vi "Update_Caliper_Overlay.vi"(5 "Analysis_Point_Result":T1[](array[typedef]), 7 "CaliperEntry":T3 {"CaliperType" items=["Distance", "Mid Point", "Perpendicular Projection", "Lines Intersection", "Angle from Horizontal", "Angle from Vertical", "Angle Defined by 3 Points", "Angle Defined by 4 Points", "Bissecting Line", "Mid Line", "Center of Mass", "Area", "Line Fit", "Circle Fit", "Ellipse Fit"]}, 11 "Image Refnum":refnum<vi>) -> ()   [LabVIEW 2019]
uses:
  Caliper/Controls/CaliperDataEntry.ctl
  Caliper/Controls/CaliperType.ctl
  Caliper/Controls/SelectionListEntry.ctl
  Caliper/Controls/SelectionListEntryPointType.ctl
  Caliper/Controls/CaliperResult.ctl
  Analysis/Controls/Analysis_Result_To_Caliper.ctl
panel:
  in  "Vision_Image":T2(plugin-control)
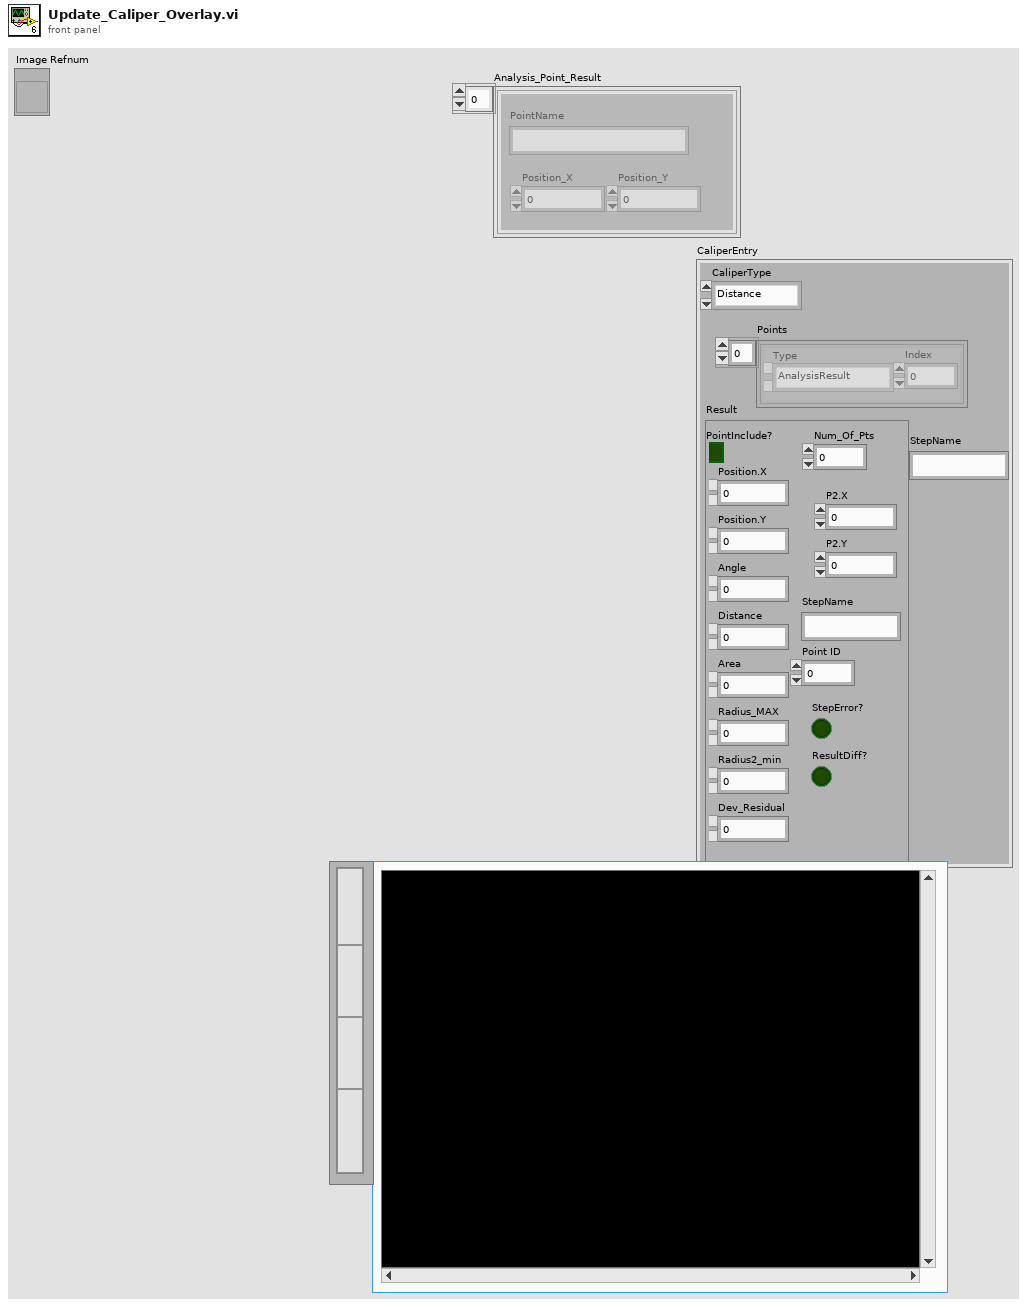
[diagram p1: front panel]
types:
  T1 = typedef "Analysis_Result_To_Caliper.ctl" = cluster{"PointName":string, "Position_X":dbl, "Position_Y":dbl}
  T2 = typedef "IMAQ Image.ctl" = refnum<image>
  T3 = typedef "CaliperDataEntry.ctl" = cluster{"CaliperType":T4, "Points":T5[], "Result":T7, "StepName":string}
  T4 = typedef "CaliperType.ctl" = u32
  T5 = typedef "SelectionListEntry.ctl" = cluster{"Type":T6, "Index":i32}
  T6 = typedef "SelectionListEntryPointType.ctl" = enum16{"AnalysisResult", "CaliperResult"}
  T7 = typedef "CaliperResult.ctl" = cluster{"PointInclude?":bool, "Num_Of_Pts":u8, "Position.X":dbl, "Position.Y":dbl, "Angle":dbl, "Distance":dbl, "Area":dbl, "Radius_MAX":dbl, "Radius2_min":dbl, "Dev_Residual":dbl, "P2.X":dbl, "P2.Y":dbl, "StepName":string, "Point ID":u8, "StepError?":bool, "ResultDiff?":bool}
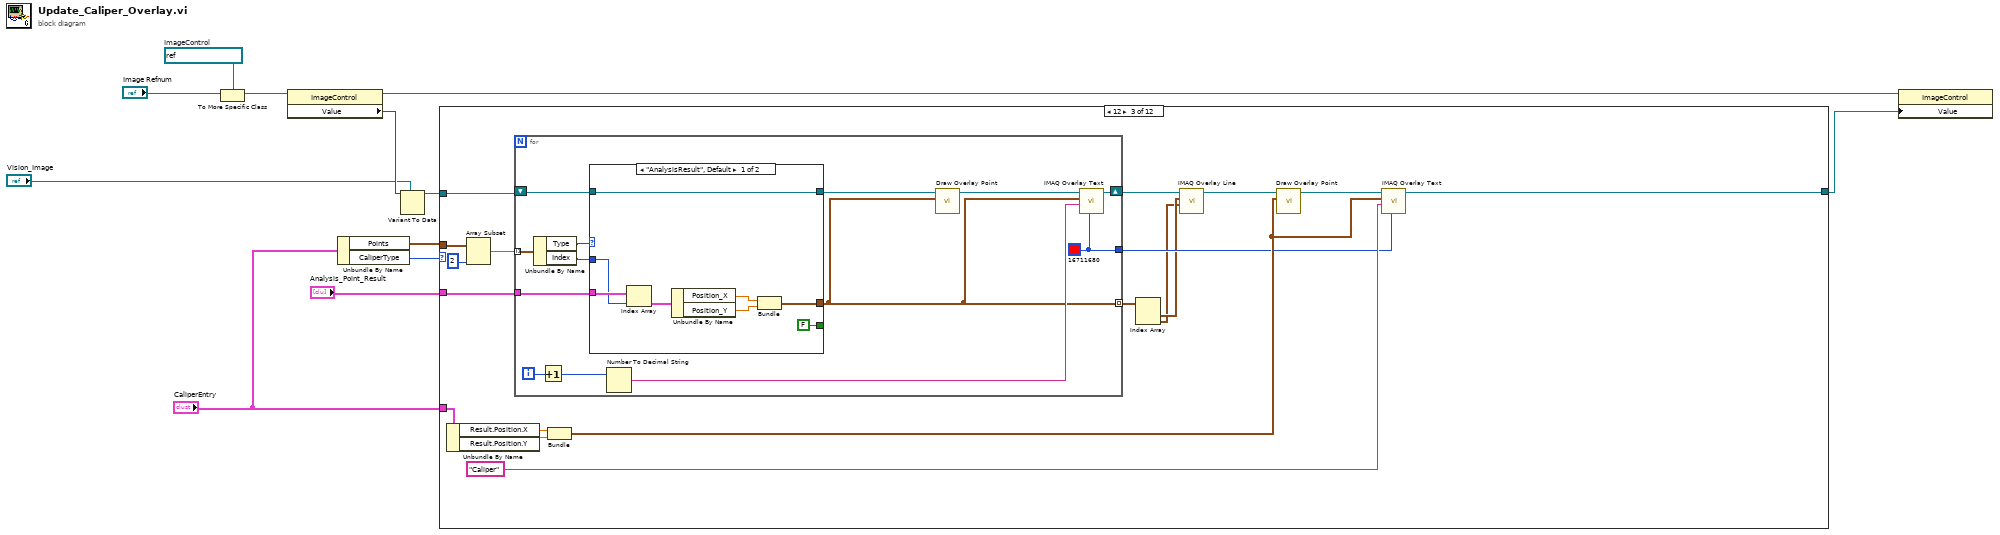
[diagram p0: block diagram]
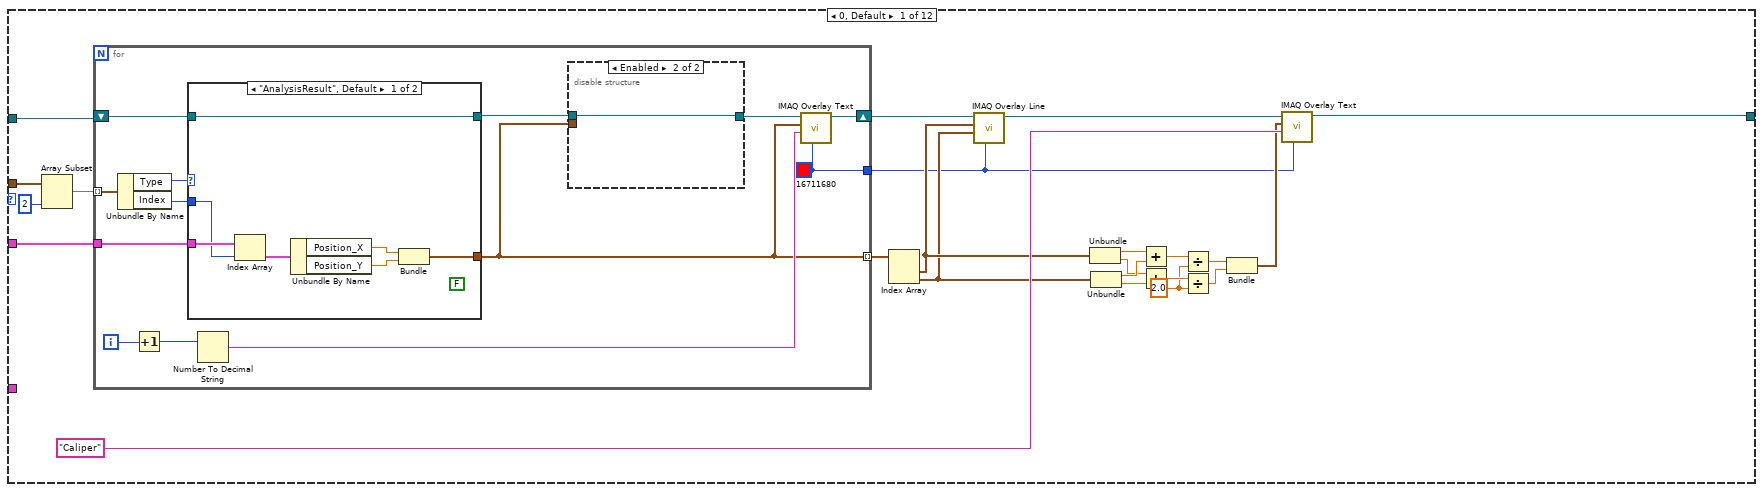
[diagram p2: hidden frame]
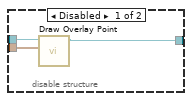
[diagram p3: hidden frame]
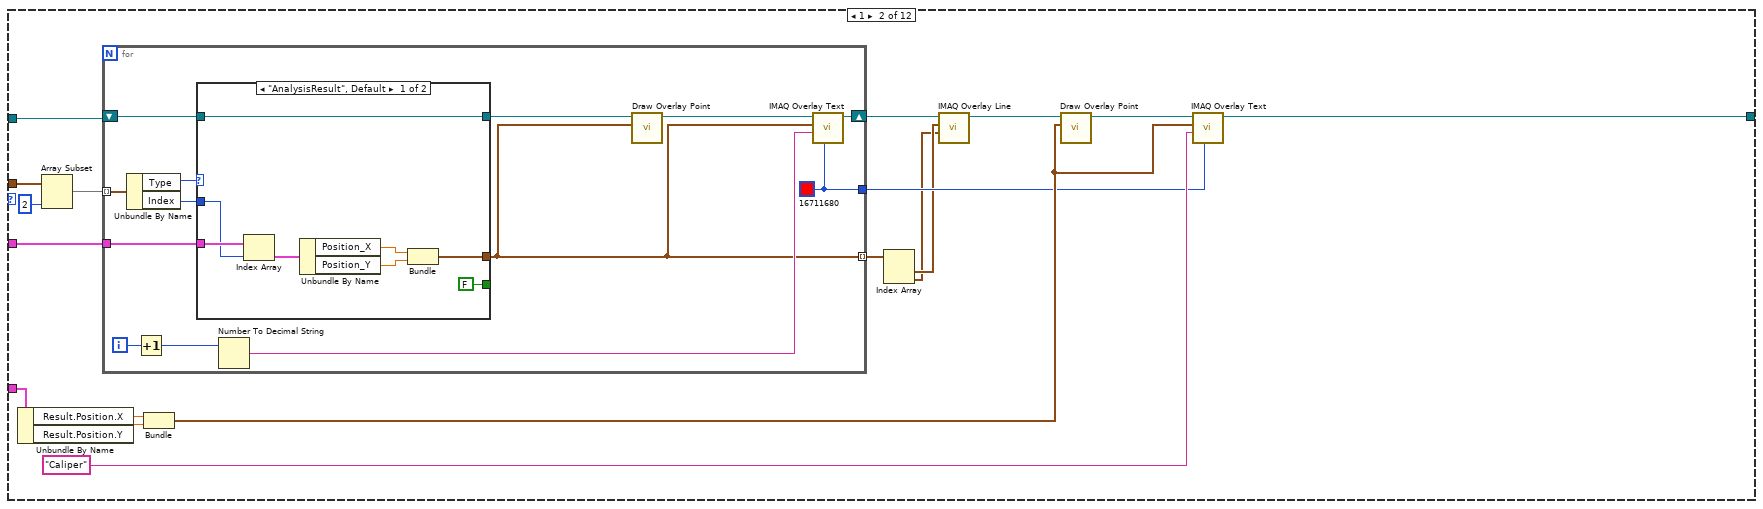
[diagram p5: hidden frame]
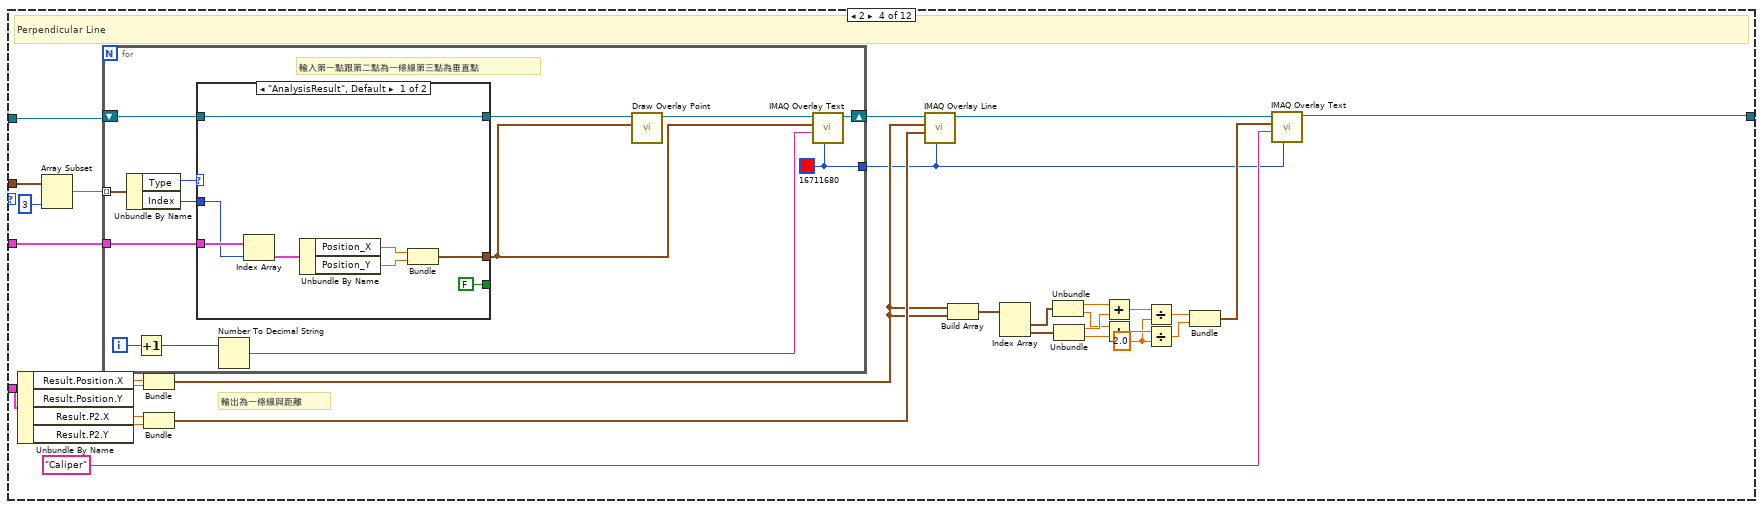
[diagram p8: hidden frame]
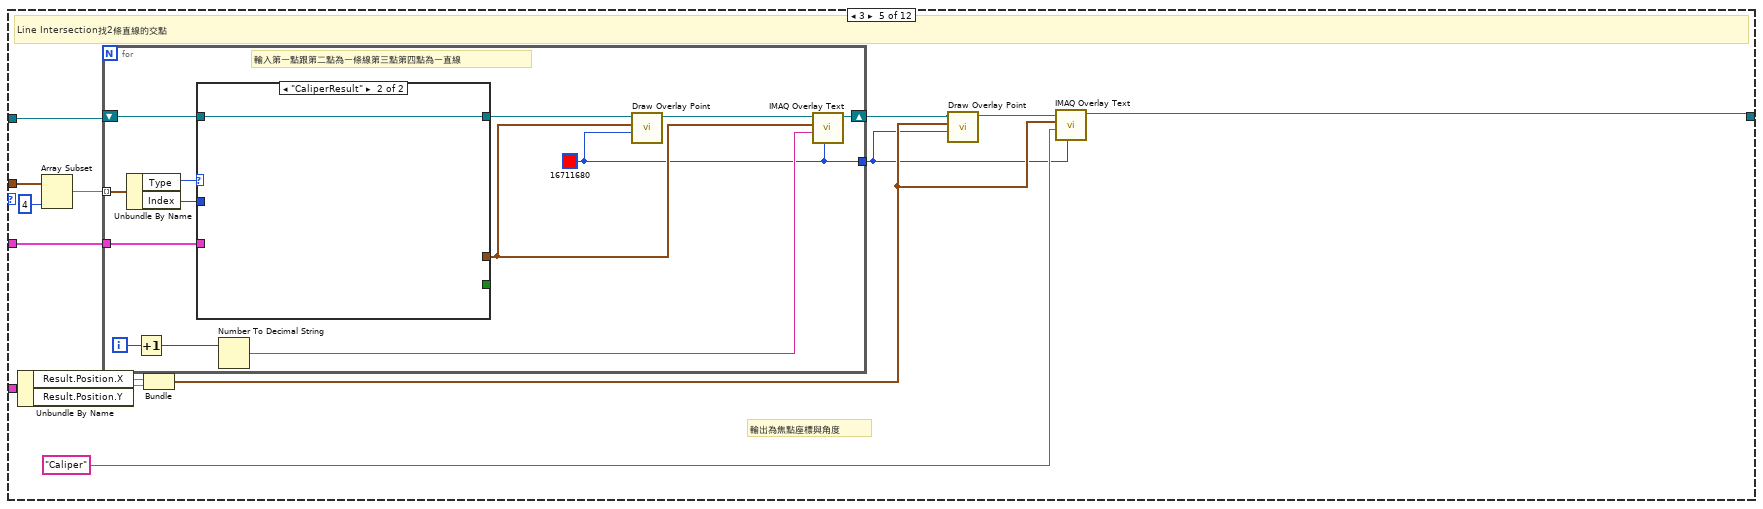
[diagram p10: hidden frame]
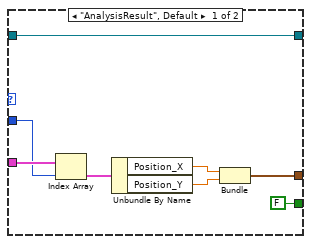
[diagram p11: hidden frame]
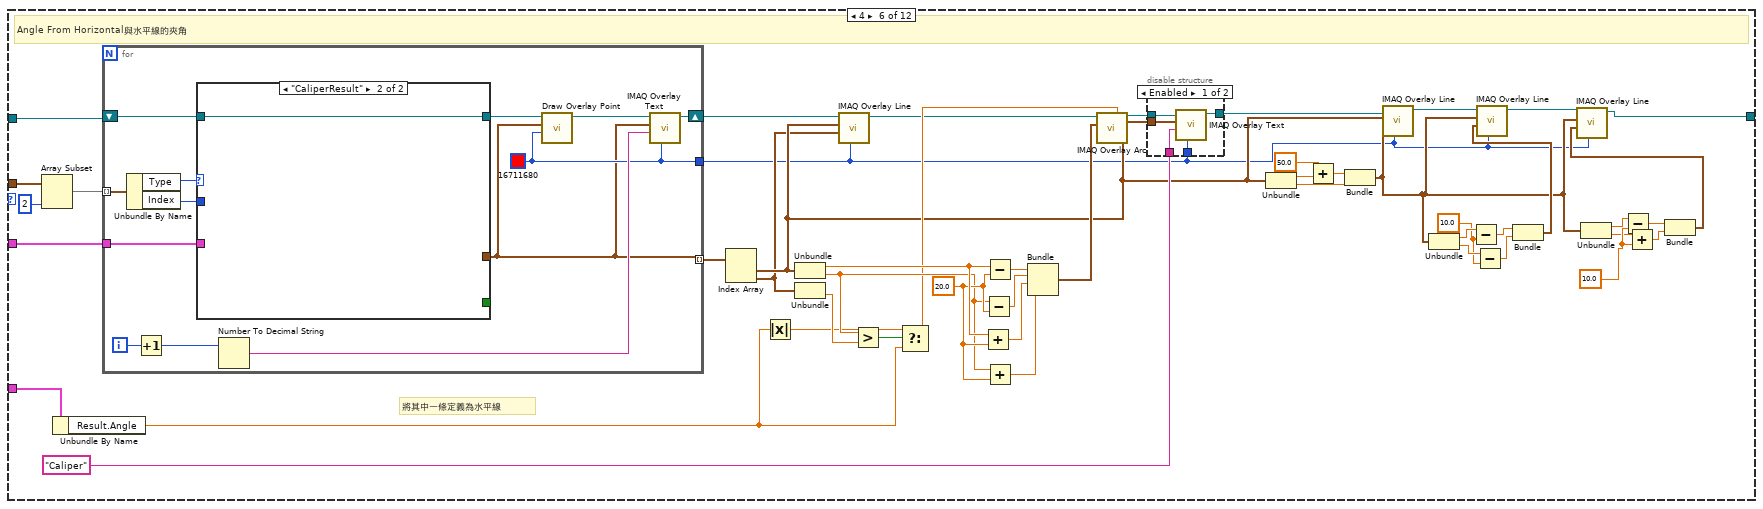
[diagram p12: hidden frame]
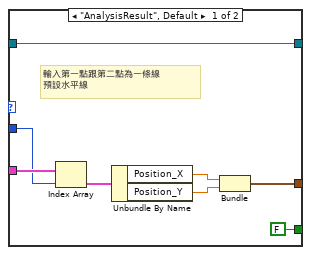
[diagram p14: hidden frame]
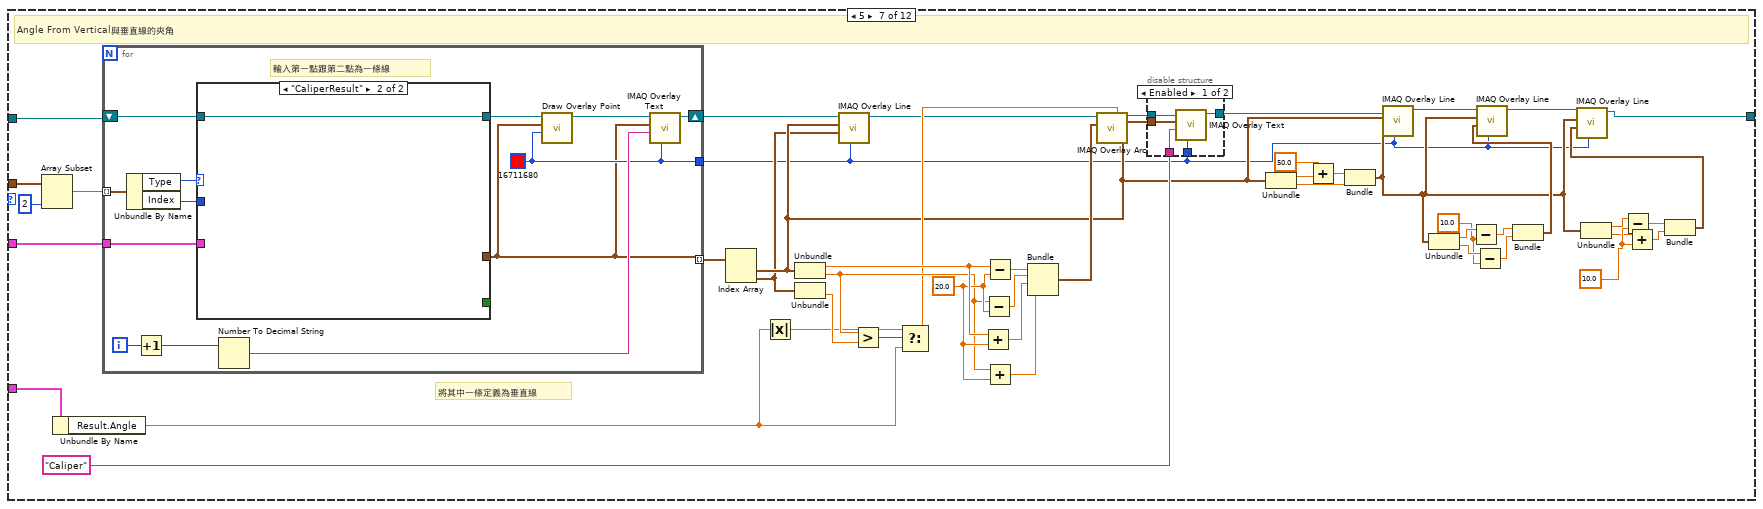
[diagram p15: hidden frame]
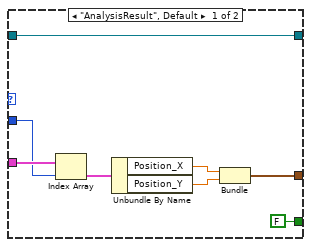
[diagram p17: hidden frame]
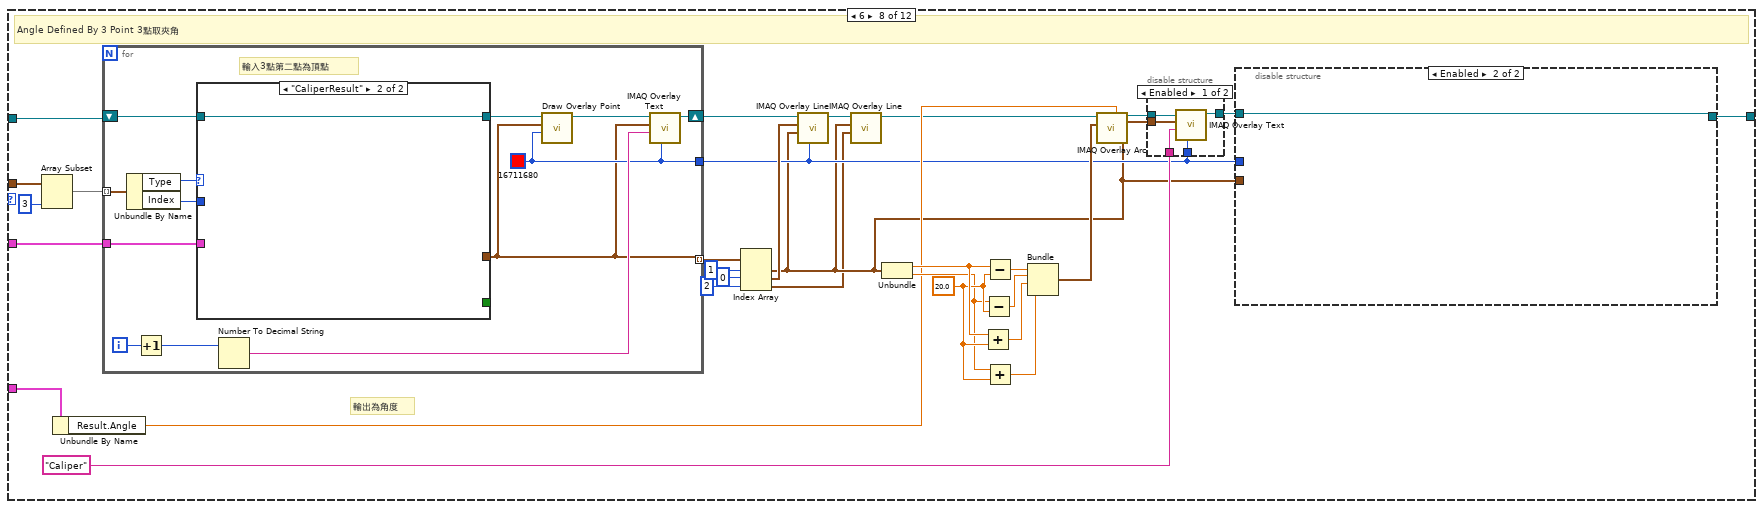
[diagram p18: hidden frame]
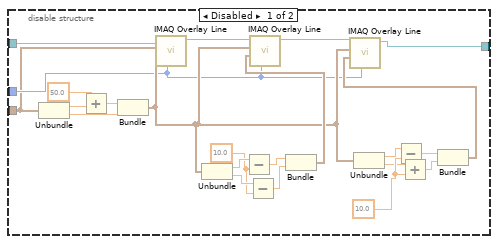
[diagram p19: hidden frame]
diagram:
  w11 = refnum<vi> refnum  # ImageControl
  n1 = To More Specific Class(target class=w11, reference="Image Refnum") -> (specific class reference=w10:refnum<vi>)  [unwired: 1 in, 1 out]
  n2 = property class="ImageControl"(reference=w10) -> (reference out=w7:refnum<vi>, "Value"=w9:variant)  [unwired: 1 in, 1 out]
  n3 = Unbundle By Name("CaliperEntry") -> ("Points"=w2:T5[], "CaliperType"=w1:T4)
  n4 = Variant To Data(type="Vision_Image", Variant=w9) -> (data=w5:T2)  [unwired: 1 in, 1 out]
  n5 = case shown="12" w1 {
    tunnel: w2 -> [w33 w76 w116 w168 w204 w274 w350 w408 w477 w535 w593 w648]
    tunnel: "Analysis_Point_Result" -> [w32 w75 w115 w167 w203 w273 w349 w407 w476 w534 w592 w647]
    tunnel: w5 -> [w31 w66 w106 w163 w201 w271 w347 w405 w474 w532 w590 w645]
    tunnel: [w29 w69 w109 w157 w196 w252 w328 w393 w464 w520 w578 w635] -> w6
    tunnel: "CaliperEntry" -> [_ w74 w114 w166 w202 w272 w348 w406 w475 w533 w591 w646]
    frame 0, Default {
      w20 = 2.0 ("y")
      n6 = Array Subset(array=w33, length=2) -> (w34:T5[])  [unwired: 1 in]
      n7 = for {
        tunnel: w34 -> [w48] mode=indexing
        tunnel: w32 -> [w46]
        shift-right: [w43] -> w30
        shift-left: w31 -> [w44]
        tunnel: [w37] -> w21 mode=indexing
        tunnel: [w36] -> w13
        i -> [w42]
        w36 = u32 16711680 ("Text Color (black)")
        n8 = Unbundle By Name(w48) -> ("Type"=w47:T6, "Index"=w45:i32)
        n9 = Increment(x=w42) -> (x+1=w41:i32)
        n10 = case shown="\"AnalysisResult\", Default" w47 {
          tunnel: w46 -> [w59 _]
          tunnel: w45 -> [w58 _]
          tunnel: [w54 _] -> w37
          tunnel: w44 -> [w53 w60]
          tunnel: [w53 w60] -> w39
          frame "AnalysisResult", Default {
            (unwired) FALSE ("StepError?")
            n11 = Index Array(array=w59, index=w58) -> (element=w57:T1)
            n12 = Unbundle By Name(w57) -> ("Position_X"=w56:dbl, "Position_Y"=w55:dbl)
            n13 = Bundle("Position_X"=w56, "Position_Y"=w55) -> (w54:cluster{"Position_X":dbl, "Position_Y":dbl})  [unwired: 1 in]
          }
          frame "CaliperResult" {
          }
        }
        n14 = Number To Decimal String(number=w41) -> (decimal integer string=w40:string)  [unwired: 1 in]
        n15 = disable-structure shown="Enabled" {
          disable-tunnel: w39 -> [w51 w52]
          disable-tunnel: [w50 w52] -> w38
          disable-tunnel: w37 -> [w49 _]
          frame Disabled {
            n16 = call "Draw Overlay Point.vi"("Cluster"=w49, "Refnum in"=w51) -> ("Refnum out"=w50:T2)  [unwired: 9 in]
          }
          frame Enabled {
          }
        }
        n17 = call "IMAQ Overlay Text"("Text Color (black)"=w36, "String"=w40, "Origin"=w37, "Image"=w38) -> ("Image Out"=w43:T2)  [unwired: 6 in, 1 out]
      }
      n18 = Index Array(array=w21) -> (element #1=w15:cluster{"Position_X":dbl, "Position_Y":dbl}, element #2=w14:cluster{"Position_X":dbl, "Position_Y":dbl})  [unwired: 2 in]
      n19 = call "IMAQ Overlay Line"("Color"=w13, "End Point"=w14, "Start Point"=w15, "Image"=w30) -> ("Image Out"=w16:T2)  [unwired: 6 in, 1 out]
      n20 = Unbundle(w15) -> ("Position_X"=w27:dbl, "Position_Y"=w24:dbl)
      n21 = Unbundle(w14) -> ("Position_X"=w25:dbl, "Position_Y"=w26:dbl)
      n22 = Add(x=w27, y=w25) -> (x+y=w23:dbl)
      n23 = Add(x=w24, y=w26) -> (x+y=w22:dbl)
      n24 = Divide(x=w23, y=w20) -> (x/y=w19:dbl)
      n25 = Divide(x=w22, y=w20) -> (x/y=w18:dbl)
      n26 = Bundle(w19, w18) -> (w17:cluster{dbl, dbl})  [unwired: 1 in]
      n27 = call "IMAQ Overlay Text"("Text Color (black)"=w13, "String"="Caliper", "Origin"=w17, "Image"=w16) -> ("Image Out"=w29:T2)  [unwired: 6 in, 1 out]
    }
    frame 1 {
      n28 = Unbundle By Name(w74) -> ("Result.Position.X"=w73:dbl, "Result.Position.Y"=w72:dbl)
      n29 = Array Subset(array=w76, length=2) -> (w77:T5[])  [unwired: 1 in]
      n30 = for {
        tunnel: w77 -> [w91] mode=indexing
        tunnel: w75 -> [w89]
        shift-right: [w84] -> w71
        shift-left: w66 -> [w87]
        tunnel: [w80] -> w65
        tunnel: [w79] -> w63 mode=indexing
        i -> [w83]
        w80 = u32 16711680 ("Text Color (black)")
        n31 = Unbundle By Name(w91) -> ("Type"=w90:T6, "Index"=w88:i32)
        n32 = Increment(x=w83) -> (x+1=w81:i32)
        n33 = case shown="\"AnalysisResult\", Default" w90 {
          tunnel: w89 -> [w99 _]
          tunnel: w88 -> [w98 _]
          tunnel: [w94 _] -> w79
          tunnel: [FALSE ("StepError?") _] -> _
          tunnel: w87 -> [w92 w100]
          tunnel: [w92 w100] -> w86
          frame "AnalysisResult", Default {
            n34 = Index Array(array=w99, index=w98) -> (element=w97:T1)
            n35 = Unbundle By Name(w97) -> ("Position_X"=w96:dbl, "Position_Y"=w95:dbl)
            n36 = Bundle("Position_X"=w96, "Position_Y"=w95) -> (w94:cluster{"Position_X":dbl, "Position_Y":dbl})  [unwired: 1 in]
          }
          frame "CaliperResult" {
          }
        }
        n37 = Number To Decimal String(number=w81) -> (decimal integer string=w82:string)  [unwired: 1 in]
        n38 = call "Draw Overlay Point.vi"("Cluster"=w79, "Refnum in"=w86) -> ("Refnum out"=w85:T2)  [unwired: 9 in]
        n39 = call "IMAQ Overlay Text"("Text Color (black)"=w80, "String"=w82, "Origin"=w79, "Image"=w85) -> ("Image Out"=w84:T2)  [unwired: 6 in, 1 out]
      }
      n40 = Bundle("Position.X"=w73, "Position.Y"=w72) -> (w68:cluster{"Position.X":dbl, "Position.Y":dbl})  [unwired: 1 in]
      n41 = Index Array(array=w63) -> (element #1=w62:cluster{"Position_X":dbl, "Position_Y":dbl}, element #2=w61:cluster{"Position_X":dbl, "Position_Y":dbl})  [unwired: 2 in]
      n42 = call "IMAQ Overlay Line"("End Point"=w61, "Start Point"=w62, "Image"=w71) -> ("Image Out"=w64:T2)  [unwired: 7 in, 1 out]
      n43 = call "Draw Overlay Point.vi"("Cluster"=w68, "Refnum in"=w64) -> ("Refnum out"=w70:T2)  [unwired: 9 in]
      n44 = call "IMAQ Overlay Text"("Text Color (black)"=w65, "String"="Caliper", "Origin"=w68, "Image"=w70) -> ("Image Out"=w69:T2)  [unwired: 6 in, 1 out]
    }
    frame 12 {
      n45 = Unbundle By Name(w114) -> ("Result.Position.X"=w113:dbl, "Result.Position.Y"=w112:dbl)
      n46 = Array Subset(array=w116, length=2) -> (w117:T5[])  [unwired: 1 in]
      n47 = for {
        tunnel: w117 -> [w131] mode=indexing
        tunnel: w115 -> [w129]
        shift-right: [w124] -> w111
        shift-left: w106 -> [w127]
        tunnel: [w120] -> w105
        tunnel: [w119] -> w103 mode=indexing
        i -> [w123]
        w120 = u32 16711680 ("Text Color (black)")
        n48 = Unbundle By Name(w131) -> ("Type"=w130:T6, "Index"=w128:i32)
        n49 = Increment(x=w123) -> (x+1=w121:i32)
        n50 = case shown="\"AnalysisResult\", Default" w130 {
          tunnel: w129 -> [w139 _]
          tunnel: w128 -> [w138 _]
          tunnel: [w134 _] -> w119
          tunnel: [FALSE ("StepError?") _] -> _
          tunnel: w127 -> [w132 w140]
          tunnel: [w132 w140] -> w126
          frame "AnalysisResult", Default {
            n51 = Index Array(array=w139, index=w138) -> (element=w137:T1)
            n52 = Unbundle By Name(w137) -> ("Position_X"=w136:dbl, "Position_Y"=w135:dbl)
            n53 = Bundle("Position_X"=w136, "Position_Y"=w135) -> (w134:cluster{"Position_X":dbl, "Position_Y":dbl})  [unwired: 1 in]
          }
          frame "CaliperResult" {
          }
        }
        n54 = Number To Decimal String(number=w121) -> (decimal integer string=w122:string)  [unwired: 1 in]
        n55 = call "Draw Overlay Point.vi"("Cluster"=w119, "Refnum in"=w126) -> ("Refnum out"=w125:T2)  [unwired: 9 in]
        n56 = call "IMAQ Overlay Text"("Text Color (black)"=w120, "String"=w122, "Origin"=w119, "Image"=w125) -> ("Image Out"=w124:T2)  [unwired: 6 in, 1 out]
      }
      n57 = Bundle("Position.X"=w113, "Position.Y"=w112) -> (w108:cluster{"Position.X":dbl, "Position.Y":dbl})  [unwired: 1 in]
      n58 = Index Array(array=w103) -> (element #1=w102:cluster{"Position_X":dbl, "Position_Y":dbl}, element #2=w101:cluster{"Position_X":dbl, "Position_Y":dbl})  [unwired: 2 in]
      n59 = call "IMAQ Overlay Line"("End Point"=w101, "Start Point"=w102, "Image"=w111) -> ("Image Out"=w104:T2)  [unwired: 7 in, 1 out]
      n60 = call "Draw Overlay Point.vi"("Cluster"=w108, "Refnum in"=w104) -> ("Refnum out"=w110:T2)  [unwired: 9 in]
      n61 = call "IMAQ Overlay Text"("Text Color (black)"=w105, "String"="Caliper", "Origin"=w108, "Image"=w110) -> ("Image Out"=w109:T2)  [unwired: 6 in, 1 out]
    }
    frame 2 {
      w147 = 2.0 ("y")
      # "輸出為一條線與距離"
      # "Perpendicular Line"
      n62 = Unbundle By Name(w166) -> ("Result.Position.X"=w162:dbl, "Result.Position.Y"=w161:dbl, "Result.P2.X"=w165:dbl, "Result.P2.Y"=w164:dbl)
      n63 = Array Subset(array=w168, length=3) -> (w169:T5[])  [unwired: 1 in]
      n64 = for {
        tunnel: w169 -> [w183] mode=indexing
        tunnel: w167 -> [w181]
        shift-right: [w176] -> w160
        shift-left: w163 -> [w179]
        tunnel: [w171] -> w141
        i -> [w174]
        w171 = u32 16711680 ("Text Color (black)")
        # "輸入第一點跟第二點為一條線第三點為垂直點"
        n65 = Unbundle By Name(w183) -> ("Type"=w182:T6, "Index"=w180:i32)
        n66 = Increment(x=w174) -> (x+1=w172:i32)
        n67 = case shown="\"AnalysisResult\", Default" w182 {
          tunnel: w181 -> [w191 _]
          tunnel: w180 -> [w190 _]
          tunnel: [w186 _] -> w175
          tunnel: [FALSE ("StepError?") _] -> _
          tunnel: w179 -> [w184 w192]
          tunnel: [w184 w192] -> w178
          frame "AnalysisResult", Default {
            n68 = Index Array(array=w191, index=w190) -> (element=w189:T1)
            n69 = Unbundle By Name(w189) -> ("Position_X"=w188:dbl, "Position_Y"=w187:dbl)
            n70 = Bundle("Position_X"=w188, "Position_Y"=w187) -> (w186:cluster{"Position_X":dbl, "Position_Y":dbl})  [unwired: 1 in]
          }
          frame "CaliperResult" {
          }
        }
        n71 = Number To Decimal String(number=w172) -> (decimal integer string=w173:string)  [unwired: 1 in]
        n72 = call "Draw Overlay Point.vi"("Cluster"=w175, "Refnum in"=w178) -> ("Refnum out"=w177:T2)  [unwired: 9 in]
        n73 = call "IMAQ Overlay Text"("Text Color (black)"=w171, "String"=w173, "Origin"=w175, "Image"=w177) -> ("Image Out"=w176:T2)  [unwired: 6 in, 1 out]
      }
      n74 = Bundle("Position.X"=w162, "Position.Y"=w161) -> (w156:cluster{"Position.X":dbl, "Position.Y":dbl})  [unwired: 1 in]
      n75 = Bundle("P2.X"=w165, "P2.Y"=w164) -> (w159:cluster{"P2.X":dbl, "P2.Y":dbl})  [unwired: 1 in]
      n76 = call "IMAQ Overlay Line"("Color"=w141, "End Point"=w159, "Start Point"=w156, "Image"=w160) -> ("Image Out"=w158:T2)  [unwired: 6 in, 1 out]
      n77 = Build Array(w156, w156) -> (w144:cluster{"Position.X":dbl, "Position.Y":dbl}[])
      n78 = Index Array(array=w144) -> (element #1=w155:cluster{"Position.X":dbl, "Position.Y":dbl}, element #2=w148:cluster{"Position.X":dbl, "Position.Y":dbl})  [unwired: 2 in]
      n79 = Unbundle(w155) -> ("Position.X"=w154:dbl, "Position.Y"=w151:dbl)
      n80 = Unbundle(w148) -> ("Position.X"=w152:dbl, "Position.Y"=w153:dbl)
      n81 = Add(x=w154, y=w152) -> (x+y=w150:dbl)
      n82 = Add(x=w151, y=w153) -> (x+y=w149:dbl)
      n83 = Divide(x=w150, y=w147) -> (x/y=w146:dbl)
      n84 = Divide(x=w149, y=w147) -> (x/y=w145:dbl)
      n85 = Bundle(w146, w145) -> (w143:cluster{dbl, dbl})  [unwired: 1 in]
      n86 = call "IMAQ Overlay Text"("Text Color (black)"=w141, "String"="Caliper", "Origin"=w143, "Image"=w158) -> ("Image Out"=w157:T2)  [unwired: 6 in, 1 out]
    }
    frame 3 {
      # "輸出為焦點座標與角度"
      # "Line Intersection找2條直線的交點"
      n87 = Unbundle By Name(w202) -> ("Result.Position.X"=w200:dbl, "Result.Position.Y"=w199:dbl)
      n88 = Array Subset(array=w204, length=4) -> (w205:T5[])  [unwired: 1 in]
      n89 = for {
        tunnel: w205 -> [w219] mode=indexing
        tunnel: w203 -> [w217]
        shift-right: [w212] -> w198
        shift-left: w201 -> [w215]
        tunnel: [w207] -> w193
        i -> [w210]
        w207 = u32 16711680 ("Text Color (black)")
        # "輸入第一點跟第二點為一條線第三點第四點為一直線"
        n90 = Unbundle By Name(w219) -> ("Type"=w218:T6, "Index"=w216:i32)
        n91 = Increment(x=w210) -> (x+1=w208:i32)
        n92 = case shown="\"CaliperResult\"" w218 {
          tunnel: w217 -> [w227 _]
          tunnel: w216 -> [w226 _]
          tunnel: [w222 _] -> w211
          tunnel: [FALSE ("StepError?") _] -> _
          tunnel: w215 -> [w220 w228]
          tunnel: [w220 w228] -> w214
          frame "AnalysisResult", Default {
            n93 = Index Array(array=w227, index=w226) -> (element=w225:T1)
            n94 = Unbundle By Name(w225) -> ("Position_X"=w224:dbl, "Position_Y"=w223:dbl)
            n95 = Bundle("Position_X"=w224, "Position_Y"=w223) -> (w222:cluster{"Position_X":dbl, "Position_Y":dbl})  [unwired: 1 in]
          }
          frame "CaliperResult" {
          }
        }
        n96 = Number To Decimal String(number=w208) -> (decimal integer string=w209:string)  [unwired: 1 in]
        n97 = call "Draw Overlay Point.vi"("Color"=w207, "Cluster"=w211, "Refnum in"=w214) -> ("Refnum out"=w213:T2)  [unwired: 8 in]
        n98 = call "IMAQ Overlay Text"("Text Color (black)"=w207, "String"=w209, "Origin"=w211, "Image"=w213) -> ("Image Out"=w212:T2)  [unwired: 6 in, 1 out]
      }
      n99 = Bundle("Position.X"=w200, "Position.Y"=w199) -> (w195:cluster{"Position.X":dbl, "Position.Y":dbl})  [unwired: 1 in]
      n100 = call "Draw Overlay Point.vi"("Color"=w193, "Cluster"=w195, "Refnum in"=w198) -> ("Refnum out"=w197:T2)  [unwired: 8 in]
      n101 = call "IMAQ Overlay Text"("Text Color (black)"=w193, "String"="Caliper", "Origin"=w195, "Image"=w197) -> ("Image Out"=w196:T2)  [unwired: 6 in, 1 out]
    }
    frame 4 {
      w240 = 10.0 ("x")
      w242 = 10.0 ("x")
      w265 = 20.0
      # "將其中一條定義為水平線"
      # "Angle From Horizontal與水平線的夾角"
      n102 = Array Subset(array=w274, length=2) -> (w275:T5[])  [unwired: 1 in]
      n103 = Unbundle By Name(w272) -> ("Result.Angle"=w234:dbl)
      n104 = for {
        tunnel: w275 -> [w295] mode=indexing
        tunnel: w273 -> [w293]
        shift-right: [w288] -> w269
        shift-left: w271 -> [w291]
        tunnel: [w284] -> w229
        tunnel: [w283] -> w267 mode=indexing
        i -> [w287]
        w284 = u32 16711680 ("Text Color (black)")
        n105 = Unbundle By Name(w295) -> ("Type"=w294:T6, "Index"=w292:i32)
        n106 = Increment(x=w287) -> (x+1=w285:i32)
        n107 = case shown="\"CaliperResult\"" w294 {
          tunnel: w293 -> [w303 _]
          tunnel: w292 -> [w302 _]
          tunnel: [w298 _] -> w283
          tunnel: [FALSE ("StepError?") _] -> _
          tunnel: w291 -> [w296 w304]
          tunnel: [w296 w304] -> w290
          frame "AnalysisResult", Default {
            # "輸入第一點跟第二點為一條線\n預設水平線"
            n108 = Index Array(array=w303, index=w302) -> (element=w301:T1)
            n109 = Unbundle By Name(w301) -> ("Position_X"=w300:dbl, "Position_Y"=w299:dbl)
            n110 = Bundle("Position_X"=w300, "Position_Y"=w299) -> (w298:cluster{"Position_X":dbl, "Position_Y":dbl})  [unwired: 1 in]
          }
          frame "CaliperResult" {
          }
        }
        n111 = Number To Decimal String(number=w285) -> (decimal integer string=w286:string)  [unwired: 1 in]
        n112 = call "Draw Overlay Point.vi"("Color"=w284, "Cluster"=w283, "Refnum in"=w290) -> ("Refnum out"=w289:T2)  [unwired: 8 in]
        n113 = call "IMAQ Overlay Text"("Text Color (black)"=w284, "String"=w286, "Origin"=w283, "Image"=w289) -> ("Image Out"=w288:T2)  [unwired: 6 in, 1 out]
      }
      n114 = Index Array(array=w267) -> (element #1=w231:cluster{"Position_X":dbl, "Position_Y":dbl}, element #2=w230:cluster{"Position_X":dbl, "Position_Y":dbl})  [unwired: 2 in]
      n115 = Absolute Value(x=w234) -> (abs(x)=w235:dbl)
      n116 = Unbundle(w231) -> ("Position_X"=w266:dbl, "Position_Y"=w238:dbl)
      n117 = Unbundle(w230) -> ("Position_Y"=w237:dbl)  [unwired: 1 out]
      n118 = call "IMAQ Overlay Line"("Color"=w229, "End Point"=w230, "Start Point"=w231, "Image"=w269) -> ("Image Out"=w232:T2)  [unwired: 6 in, 1 out]
      n119 = Greater?(x=w238, y=w237) -> (0:w236:bool)
      n120 = Select(t=w235, s=w236, f=w234) -> (s? t:f=w233:dbl)
      n121 = Add(x=w266, y=w265) -> (x+y=w262:dbl)
      n122 = Subtract(x=w238, y=w265) -> (x-y=w263:dbl)
      n123 = Subtract(x=w266, y=w265) -> (x-y=w264:dbl)
      n124 = Add(x=w238, y=w265) -> (x+y=w261:dbl)
      n125 = Bundle(w264, w263, w262, w261) -> (w260:cluster{dbl, dbl, dbl, dbl})  [unwired: 1 in]
      n126 = call "IMAQ Overlay Arc"("End Angle (degrees)"=w233, "Bounding Rectangle"=w260, "Image"=w232) -> ("Image Out"=w268:T2)  [unwired: 7 in, 1 out]
      n127 = disable-structure shown="Enabled" {
        disable-tunnel: [w281 w282] -> w259
        disable-tunnel: "Caliper" -> [w280 _]
        disable-tunnel: w229 -> [w279 _]
        disable-tunnel: w268 -> [w278 w282]
        disable-tunnel: w231 -> [w277 _]
        frame Enabled {
          n128 = call "IMAQ Overlay Text"("Text Color (black)"=w279, "String"=w280, "Origin"=w277, "Image"=w278) -> ("Image Out"=w281:T2)  [unwired: 6 in, 1 out]
        }
        frame Disabled {
        }
      }
      n129 = Unbundle(w231) -> ("Position_X"=w258:dbl, "Position_Y"=w255:dbl)
      n130 = Add(x=50.0, y=w258) -> (x+y=w256:dbl)
      n131 = Bundle(w256, "Position_Y"=w255) -> (w245:cluster{dbl, "Position_Y":dbl})  [unwired: 1 in]
      n132 = call "IMAQ Overlay Line"("Color"=w229, "End Point"=w245, "Start Point"=w231, "Image"=w259) -> ("Image Out"=w254:T2)  [unwired: 6 in, 1 out]
      n133 = Unbundle(w245) -> (w244:dbl, "Position_Y"=w243:dbl)
      n134 = Subtract(x=w244, y=w242) -> (x-y=w251:dbl)
      n135 = Subtract(x=w243, y=w242) -> (x-y=w250:dbl)
      n136 = Bundle(w251, w250) -> (w249:cluster{dbl, dbl})  [unwired: 1 in]
      n137 = call "IMAQ Overlay Line"("Color"=w229, "End Point"=w249, "Start Point"=w245, "Image"=w254) -> ("Image Out"=w253:T2)  [unwired: 6 in, 1 out]
      n138 = Unbundle(w245) -> (w241:dbl, "Position_Y"=w239:dbl)
      n139 = Subtract(x=w241, y=w240) -> (x-y=w247:dbl)
      n140 = Add(x=w239, y=w240) -> (x+y=w248:dbl)
      n141 = Bundle(w247, w248) -> (w246:cluster{dbl, dbl})  [unwired: 1 in]
      n142 = call "IMAQ Overlay Line"("Color"=w229, "End Point"=w246, "Start Point"=w245, "Image"=w253) -> ("Image Out"=w252:T2)  [unwired: 6 in, 1 out]
    }
    frame 5 {
      w316 = 10.0 ("x")
      w318 = 10.0 ("x")
      w341 = 20.0
      # "將其中一條定義為垂直線"
      # "Angle From Vertical與垂直線的夾角"
      n143 = Array Subset(array=w350, length=2) -> (w351:T5[])  [unwired: 1 in]
      n144 = Unbundle By Name(w348) -> ("Result.Angle"=w310:dbl)
      n145 = for {
        tunnel: w351 -> [w371] mode=indexing
        tunnel: w349 -> [w369]
        shift-right: [w364] -> w345
        shift-left: w347 -> [w367]
        tunnel: [w360] -> w305
        tunnel: [w359] -> w343 mode=indexing
        i -> [w363]
        w360 = u32 16711680 ("Text Color (black)")
        # "輸入第一點跟第二點為一條線"
        n146 = Unbundle By Name(w371) -> ("Type"=w370:T6, "Index"=w368:i32)
        n147 = Increment(x=w363) -> (x+1=w361:i32)
        n148 = case shown="\"CaliperResult\"" w370 {
          tunnel: w369 -> [w379 _]
          tunnel: w368 -> [w378 _]
          tunnel: [w374 _] -> w359
          tunnel: [FALSE ("StepError?") _] -> _
          tunnel: w367 -> [w372 w380]
          tunnel: [w372 w380] -> w366
          frame "AnalysisResult", Default {
            n149 = Index Array(array=w379, index=w378) -> (element=w377:T1)
            n150 = Unbundle By Name(w377) -> ("Position_X"=w376:dbl, "Position_Y"=w375:dbl)
            n151 = Bundle("Position_X"=w376, "Position_Y"=w375) -> (w374:cluster{"Position_X":dbl, "Position_Y":dbl})  [unwired: 1 in]
          }
          frame "CaliperResult" {
          }
        }
        n152 = Number To Decimal String(number=w361) -> (decimal integer string=w362:string)  [unwired: 1 in]
        n153 = call "Draw Overlay Point.vi"("Color"=w360, "Cluster"=w359, "Refnum in"=w366) -> ("Refnum out"=w365:T2)  [unwired: 8 in]
        n154 = call "IMAQ Overlay Text"("Text Color (black)"=w360, "String"=w362, "Origin"=w359, "Image"=w365) -> ("Image Out"=w364:T2)  [unwired: 6 in, 1 out]
      }
      n155 = Index Array(array=w343) -> (element #1=w307:cluster{"Position_X":dbl, "Position_Y":dbl}, element #2=w306:cluster{"Position_X":dbl, "Position_Y":dbl})  [unwired: 2 in]
      n156 = Absolute Value(x=w310) -> (abs(x)=w311:dbl)
      n157 = Unbundle(w307) -> ("Position_X"=w342:dbl, "Position_Y"=w314:dbl)
      n158 = Unbundle(w306) -> ("Position_Y"=w313:dbl)  [unwired: 1 out]
      n159 = call "IMAQ Overlay Line"("Color"=w305, "End Point"=w306, "Start Point"=w307, "Image"=w345) -> ("Image Out"=w308:T2)  [unwired: 6 in, 1 out]
      n160 = Greater?(x=w314, y=w313) -> (0:w312:bool)
      n161 = Select(t=w311, s=w312, f=w310) -> (s? t:f=w309:dbl)
      n162 = Add(x=w342, y=w341) -> (x+y=w338:dbl)
      n163 = Subtract(x=w314, y=w341) -> (x-y=w339:dbl)
      n164 = Subtract(x=w342, y=w341) -> (x-y=w340:dbl)
      n165 = Add(x=w314, y=w341) -> (x+y=w337:dbl)
      n166 = Bundle(w340, w339, w338, w337) -> (w336:cluster{dbl, dbl, dbl, dbl})  [unwired: 1 in]
      n167 = call "IMAQ Overlay Arc"("End Angle (degrees)"=w309, "Bounding Rectangle"=w336, "Image"=w308) -> ("Image Out"=w344:T2)  [unwired: 7 in, 1 out]
      n168 = disable-structure shown="Enabled" {
        disable-tunnel: [w357 w358] -> w335
        disable-tunnel: "Caliper" -> [w356 _]
        disable-tunnel: w305 -> [w355 _]
        disable-tunnel: w344 -> [w354 w358]
        disable-tunnel: w307 -> [w353 _]
        frame Enabled {
          n169 = call "IMAQ Overlay Text"("Text Color (black)"=w355, "String"=w356, "Origin"=w353, "Image"=w354) -> ("Image Out"=w357:T2)  [unwired: 6 in, 1 out]
        }
        frame Disabled {
        }
      }
      n170 = Unbundle(w307) -> ("Position_X"=w334:dbl, "Position_Y"=w331:dbl)
      n171 = Add(x=50.0, y=w334) -> (x+y=w332:dbl)
      n172 = Bundle(w332, "Position_Y"=w331) -> (w321:cluster{dbl, "Position_Y":dbl})  [unwired: 1 in]
      n173 = call "IMAQ Overlay Line"("Color"=w305, "End Point"=w321, "Start Point"=w307, "Image"=w335) -> ("Image Out"=w330:T2)  [unwired: 6 in, 1 out]
      n174 = Unbundle(w321) -> (w320:dbl, "Position_Y"=w319:dbl)
      n175 = Subtract(x=w320, y=w318) -> (x-y=w327:dbl)
      n176 = Subtract(x=w319, y=w318) -> (x-y=w326:dbl)
      n177 = Bundle(w327, w326) -> (w325:cluster{dbl, dbl})  [unwired: 1 in]
      n178 = call "IMAQ Overlay Line"("Color"=w305, "End Point"=w325, "Start Point"=w321, "Image"=w330) -> ("Image Out"=w329:T2)  [unwired: 6 in, 1 out]
      n179 = Unbundle(w321) -> (w317:dbl, "Position_Y"=w315:dbl)
      n180 = Subtract(x=w317, y=w316) -> (x-y=w323:dbl)
      n181 = Add(x=w315, y=w316) -> (x+y=w324:dbl)
      n182 = Bundle(w323, w324) -> (w322:cluster{dbl, dbl})  [unwired: 1 in]
      n183 = call "IMAQ Overlay Line"("Color"=w305, "End Point"=w322, "Start Point"=w321, "Image"=w329) -> ("Image Out"=w328:T2)  [unwired: 6 in, 1 out]
    }
    frame 6 {
      w400 = 20.0
      # "輸出為角度"
      # "Angle Defined By 3 Point 3點取夾角"
      n184 = Array Subset(array=w408, length=3) -> (w409:T5[])  [unwired: 1 in]
      n185 = Unbundle By Name(w406) -> ("Result.Angle"=w390:dbl)
      n186 = for {
        tunnel: w409 -> [w453] mode=indexing
        tunnel: w407 -> [w451]
        shift-right: [w446] -> w391
        shift-left: w405 -> [w449]
        tunnel: [w442] -> w384
        tunnel: [w441] -> w402 mode=indexing
        i -> [w445]
        w442 = u32 16711680 ("Text Color (black)")
        # "輸入3點第二點為頂點"
        n187 = Unbundle By Name(w453) -> ("Type"=w452:T6, "Index"=w450:i32)
        n188 = Increment(x=w445) -> (x+1=w443:i32)
        n189 = case shown="\"CaliperResult\"" w452 {
          tunnel: w451 -> [w461 _]
          tunnel: w450 -> [w460 _]
          tunnel: [w456 _] -> w441
          tunnel: [FALSE ("StepError?") _] -> _
          tunnel: w449 -> [w454 w462]
          tunnel: [w454 w462] -> w448
          frame "AnalysisResult", Default {
            n190 = Index Array(array=w461, index=w460) -> (element=w459:T1)
            n191 = Unbundle By Name(w459) -> ("Position_X"=w458:dbl, "Position_Y"=w457:dbl)
            n192 = Bundle("Position_X"=w458, "Position_Y"=w457) -> (w456:cluster{"Position_X":dbl, "Position_Y":dbl})  [unwired: 1 in]
          }
          frame "CaliperResult" {
          }
        }
        n193 = Number To Decimal String(number=w443) -> (decimal integer string=w444:string)  [unwired: 1 in]
        n194 = call "Draw Overlay Point.vi"("Color"=w442, "Cluster"=w441, "Refnum in"=w448) -> ("Refnum out"=w447:T2)  [unwired: 8 in]
        n195 = call "IMAQ Overlay Text"("Text Color (black)"=w442, "String"=w444, "Origin"=w441, "Image"=w447) -> ("Image Out"=w446:T2)  [unwired: 6 in, 1 out]
      }
      n196 = Index Array(array=w402, index #1=1 ("index"), index #2=0 ("index"), index #3=2 ("index")) -> (element #1=w382:cluster{"Position_X":dbl, "Position_Y":dbl}, element #2=w385:cluster{"Position_X":dbl, "Position_Y":dbl}, element #3=w381:cluster{"Position_X":dbl, "Position_Y":dbl})
      n197 = call "IMAQ Overlay Line"("Color"=w384, "End Point"=w382, "Start Point"=w385, "Image"=w391) -> ("Image Out"=w388:T2)  [unwired: 6 in, 1 out]
      n198 = call "IMAQ Overlay Line"("End Point"=w381, "Start Point"=w382, "Image"=w388) -> ("Image Out"=w383:T2)  [unwired: 7 in, 1 out]
      n199 = Unbundle(w382) -> ("Position_X"=w401:dbl, "Position_Y"=w392:dbl)
      n200 = Add(x=w401, y=w400) -> (x+y=w397:dbl)
      n201 = Subtract(x=w392, y=w400) -> (x-y=w398:dbl)
      n202 = Subtract(x=w401, y=w400) -> (x-y=w399:dbl)
      n203 = Add(x=w392, y=w400) -> (x+y=w396:dbl)
      n204 = Bundle(w399, w398, w397, w396) -> (w395:cluster{dbl, dbl, dbl, dbl})  [unwired: 1 in]
      n205 = call "IMAQ Overlay Arc"("End Angle (degrees)"=w390, "Bounding Rectangle"=w395, "Image"=w383) -> ("Image Out"=w403:T2)  [unwired: 7 in, 1 out]
      n206 = disable-structure shown="Enabled" {
        disable-tunnel: [w439 w440] -> w394
        disable-tunnel: "Caliper" -> [w438 _]
        disable-tunnel: w384 -> [w437 _]
        disable-tunnel: w403 -> [w436 w440]
        disable-tunnel: w382 -> [w435 _]
        frame Enabled {
          n207 = call "IMAQ Overlay Text"("Text Color (black)"=w437, "String"=w438, "Origin"=w435, "Image"=w436) -> ("Image Out"=w439:T2)  [unwired: 6 in, 1 out]
        }
        frame Disabled {
        }
      }
      n208 = disable-structure shown="Enabled" {
        disable-tunnel: w394 -> [w433 w434]
        disable-tunnel: [w426 w434] -> w393
        disable-tunnel: w384 -> [w412 _]
        disable-tunnel: w382 -> [w411 _]
        frame Disabled {
          w414 = 10.0 ("x")
          w416 = 10.0 ("x")
          n209 = Unbundle(w411) -> ("Position_X"=w432:dbl, "Position_Y"=w429:dbl)
          n210 = Add(x=50.0, y=w432) -> (x+y=w430:dbl)
          n211 = Bundle(w430, "Position_Y"=w429) -> (w419:cluster{dbl, "Position_Y":dbl})  [unwired: 1 in]
          n212 = call "IMAQ Overlay Line"("Color"=w412, "End Point"=w419, "Start Point"=w411, "Image"=w433) -> ("Image Out"=w428:T2)  [unwired: 6 in, 1 out]
          n213 = Unbundle(w419) -> (w418:dbl, "Position_Y"=w417:dbl)
          n214 = Subtract(x=w418, y=w416) -> (x-y=w425:dbl)
          n215 = Subtract(x=w417, y=w416) -> (x-y=w424:dbl)
          n216 = Bundle(w425, w424) -> (w423:cluster{dbl, dbl})  [unwired: 1 in]
          n217 = call "IMAQ Overlay Line"("Color"=w412, "End Point"=w423, "Start Point"=w419, "Image"=w428) -> ("Image Out"=w427:T2)  [unwired: 6 in, 1 out]
          n218 = Unbundle(w419) -> (w415:dbl, "Position_Y"=w413:dbl)
          n219 = Subtract(x=w415, y=w414) -> (x-y=w421:dbl)
          n220 = Add(x=w413, y=w414) -> (x+y=w422:dbl)
          n221 = Bundle(w421, w422) -> (w420:cluster{dbl, dbl})  [unwired: 1 in]
          n222 = call "IMAQ Overlay Line"("Color"=w412, "End Point"=w420, "Start Point"=w419, "Image"=w427) -> ("Image Out"=w426:T2)  [unwired: 6 in, 1 out]
        }
        frame Enabled {
        }
      }
    }
    frame 7 {
      (unwired) "Caliper"
      n223 = Array Subset(array=w477, length=3) -> (w478:T5[])  [unwired: 1 in]
      n224 = Unbundle By Name(w475) -> ()  [unwired: 1 out]
      n225 = for {
        tunnel: w478 -> [w492] mode=indexing
        tunnel: w476 -> [w490]
        shift-right: [w485] -> w472
        shift-left: w474 -> [w488]
        tunnel: [w481] -> w463
        tunnel: [w480] -> w473 mode=indexing
        i -> [w484]
        w481 = u32 16711680 ("Text Color (black)")
        n226 = Unbundle By Name(w492) -> ("Type"=w491:T6, "Index"=w489:i32)
        n227 = Increment(x=w484) -> (x+1=w482:i32)
        n228 = case shown="\"CaliperResult\"" w491 {
          tunnel: w490 -> [w500 _]
          tunnel: w489 -> [w499 _]
          tunnel: [w495 _] -> w480
          tunnel: [FALSE ("StepError?") _] -> _
          tunnel: w488 -> [w493 w501]
          tunnel: [w493 w501] -> w487
          frame "AnalysisResult", Default {
            n229 = Index Array(array=w500, index=w499) -> (element=w498:T1)
            n230 = Unbundle By Name(w498) -> ("Position_X"=w497:dbl, "Position_Y"=w496:dbl)
            n231 = Bundle("Position_X"=w497, "Position_Y"=w496) -> (w495:cluster{"Position_X":dbl, "Position_Y":dbl})  [unwired: 1 in]
          }
          frame "CaliperResult" {
          }
        }
        n232 = Number To Decimal String(number=w482) -> (decimal integer string=w483:string)  [unwired: 1 in]
        n233 = call "Draw Overlay Point.vi"("Color"=w481, "Cluster"=w480, "Refnum in"=w487) -> ("Refnum out"=w486:T2)  [unwired: 8 in]
        n234 = call "IMAQ Overlay Text"("Text Color (black)"=w481, "String"=w483, "Origin"=w480, "Image"=w486) -> ("Image Out"=w485:T2)  [unwired: 6 in, 1 out]
      }
      n235 = Index Array(array=w473, index #1=1 ("index"), index #2=0 ("index"), index #3=2 ("index")) -> (element #1=w466:cluster{"Position_X":dbl, "Position_Y":dbl}, element #2=w467:cluster{"Position_X":dbl, "Position_Y":dbl}, element #3=w465:cluster{"Position_X":dbl, "Position_Y":dbl})
      n236 = call "IMAQ Overlay Line"("Color"=w463, "End Point"=w466, "Start Point"=w467, "Image"=w472) -> ("Image Out"=w470:T2)  [unwired: 6 in, 1 out]
      n237 = call "IMAQ Overlay Line"("Color"=w463, "End Point"=w465, "Start Point"=w466, "Image"=w470) -> ("Image Out"=w464:T2)  [unwired: 6 in, 1 out]
    }
    frame 8 {
      w511 = 2.0 ("y")
      n238 = Unbundle By Name(w533) -> ("Result.Position.X"=w526:dbl, "Result.Position.Y"=w525:dbl, "Result.P2.X"=w524:dbl, "Result.P2.Y"=w523:dbl)
      n239 = Array Subset(array=w535, length=4) -> (w536:T5[])  [unwired: 1 in]
      n240 = for {
        tunnel: w536 -> [w550] mode=indexing
        tunnel: w534 -> [w548]
        shift-right: [w543] -> w530
        shift-left: w532 -> [w546]
        tunnel: [w539] -> w519
        tunnel: [w538] -> w531 mode=indexing
        i -> [w542]
        w539 = u32 16711680 ("Text Color (black)")
        n241 = Unbundle By Name(w550) -> ("Type"=w549:T6, "Index"=w547:i32)
        n242 = Increment(x=w542) -> (x+1=w540:i32)
        n243 = case shown="\"CaliperResult\"" w549 {
          tunnel: w548 -> [w558 _]
          tunnel: w547 -> [w557 _]
          tunnel: [w553 _] -> w538
          tunnel: [FALSE ("StepError?") _] -> _
          tunnel: w546 -> [w551 w559]
          tunnel: [w551 w559] -> w545
          frame "AnalysisResult", Default {
            n244 = Index Array(array=w558, index=w557) -> (element=w556:T1)
            n245 = Unbundle By Name(w556) -> ("Position_X"=w555:dbl, "Position_Y"=w554:dbl)
            n246 = Bundle("Position_X"=w555, "Position_Y"=w554) -> (w553:cluster{"Position_X":dbl, "Position_Y":dbl})  [unwired: 1 in]
          }
          frame "CaliperResult" {
          }
        }
        n247 = Number To Decimal String(number=w540) -> (decimal integer string=w541:string)  [unwired: 1 in]
        n248 = call "Draw Overlay Point.vi"("Color"=w539, "Cluster"=w538, "Refnum in"=w545) -> ("Refnum out"=w544:T2)  [unwired: 8 in]
        n249 = call "IMAQ Overlay Text"("Text Color (black)"=w539, "String"=w541, "Origin"=w538, "Image"=w544) -> ("Image Out"=w543:T2)  [unwired: 6 in, 1 out]
      }
      n250 = Bundle("P2.X"=w524, "P2.Y"=w523) -> (w507:cluster{"P2.X":dbl, "P2.Y":dbl})  [unwired: 1 in]
      n251 = Bundle("Position.X"=w526, "Position.Y"=w525) -> (w508:cluster{"Position.X":dbl, "Position.Y":dbl})  [unwired: 1 in]
      n252 = Index Array(array=w531) -> (element #1=w505:cluster{"Position_X":dbl, "Position_Y":dbl}, element #2=w504:cluster{"Position_X":dbl, "Position_Y":dbl}, element #3=w503:cluster{"Position_X":dbl, "Position_Y":dbl}, element #4=w502:cluster{"Position_X":dbl, "Position_Y":dbl})  [unwired: 4 in]
      n253 = call "IMAQ Overlay Line"("Color"=w519, "End Point"=w504, "Start Point"=w505, "Image"=w530) -> ("Image Out"=w529:T2)  [unwired: 6 in, 1 out]
      n254 = call "IMAQ Overlay Line"("Color"=w519, "End Point"=w502, "Start Point"=w503, "Image"=w529) -> ("Image Out"=w528:T2)  [unwired: 6 in, 1 out]
      n255 = call "Draw Overlay Point.vi"("Color"=w519, "Cluster"=w508, "Refnum in"=w528) -> ("Refnum out"=w527:T2)  [unwired: 8 in]
      n256 = call "Draw Overlay Point.vi"("Color"=w519, "Cluster"=w507, "Refnum in"=w527) -> ("Refnum out"=w522:T2)  [unwired: 8 in]
      n257 = Unbundle(w508) -> ("Position.X"=w517:dbl, "Position.Y"=w514:dbl)
      n258 = Unbundle(w507) -> ("P2.X"=w515:dbl, "P2.Y"=w516:dbl)
      n259 = Add(x=w517, y=w515) -> (x+y=w513:dbl)
      n260 = Add(x=w514, y=w516) -> (x+y=w512:dbl)
      n261 = call "IMAQ Overlay Line"("Color"=w519, "End Point"=w507, "Start Point"=w508, "Image"=w522) -> ("Image Out"=w521:T2)  [unwired: 6 in, 1 out]
      n262 = Divide(x=w513, y=w511) -> (x/y=w510:dbl)
      n263 = Divide(x=w512, y=w511) -> (x/y=w509:dbl)
      n264 = Bundle(w510, w509) -> (w506:cluster{dbl, dbl})  [unwired: 1 in]
      n265 = call "IMAQ Overlay Text"("Text Color (black)"=w519, "String"="Caliper", "Origin"=w506, "Image"=w521) -> ("Image Out"=w520:T2)  [unwired: 6 in, 1 out]
    }
    frame 11 {
      w569 = 2.0 ("y")
      n266 = Unbundle By Name(w591) -> ("Result.Position.X"=w584:dbl, "Result.Position.Y"=w583:dbl, "Result.P2.X"=w582:dbl, "Result.P2.Y"=w581:dbl)
      n267 = Array Subset(array=w593, length=4) -> (w594:T5[])  [unwired: 1 in]
      n268 = for {
        tunnel: w594 -> [w608] mode=indexing
        tunnel: w592 -> [w606]
        shift-right: [w601] -> w588
        shift-left: w590 -> [w604]
        tunnel: [w597] -> w577
        tunnel: [w596] -> w589 mode=indexing
        i -> [w600]
        w597 = u32 16711680 ("Text Color (black)")
        n269 = Unbundle By Name(w608) -> ("Type"=w607:T6, "Index"=w605:i32)
        n270 = Increment(x=w600) -> (x+1=w598:i32)
        n271 = case shown="\"CaliperResult\"" w607 {
          tunnel: w606 -> [w616 _]
          tunnel: w605 -> [w615 _]
          tunnel: [w611 _] -> w596
          tunnel: [FALSE ("StepError?") _] -> _
          tunnel: w604 -> [w609 w617]
          tunnel: [w609 w617] -> w603
          frame "AnalysisResult", Default {
            n272 = Index Array(array=w616, index=w615) -> (element=w614:T1)
            n273 = Unbundle By Name(w614) -> ("Position_X"=w613:dbl, "Position_Y"=w612:dbl)
            n274 = Bundle("Position_X"=w613, "Position_Y"=w612) -> (w611:cluster{"Position_X":dbl, "Position_Y":dbl})  [unwired: 1 in]
          }
          frame "CaliperResult" {
          }
        }
        n275 = Number To Decimal String(number=w598) -> (decimal integer string=w599:string)  [unwired: 1 in]
        n276 = call "Draw Overlay Point.vi"("Color"=w597, "Cluster"=w596, "Refnum in"=w603) -> ("Refnum out"=w602:T2)  [unwired: 8 in]
        n277 = call "IMAQ Overlay Text"("Text Color (black)"=w597, "String"=w599, "Origin"=w596, "Image"=w602) -> ("Image Out"=w601:T2)  [unwired: 6 in, 1 out]
      }
      n278 = Bundle("P2.X"=w582, "P2.Y"=w581) -> (w565:cluster{"P2.X":dbl, "P2.Y":dbl})  [unwired: 1 in]
      n279 = Bundle("Position.X"=w584, "Position.Y"=w583) -> (w566:cluster{"Position.X":dbl, "Position.Y":dbl})  [unwired: 1 in]
      n280 = Index Array(array=w589) -> (element #1=w563:cluster{"Position_X":dbl, "Position_Y":dbl}, element #2=w562:cluster{"Position_X":dbl, "Position_Y":dbl}, element #3=w561:cluster{"Position_X":dbl, "Position_Y":dbl}, element #4=w560:cluster{"Position_X":dbl, "Position_Y":dbl})  [unwired: 4 in]
      n281 = call "IMAQ Overlay Line"("Color"=w577, "End Point"=w562, "Start Point"=w563, "Image"=w588) -> ("Image Out"=w587:T2)  [unwired: 6 in, 1 out]
      n282 = call "IMAQ Overlay Line"("Color"=w577, "End Point"=w560, "Start Point"=w561, "Image"=w587) -> ("Image Out"=w586:T2)  [unwired: 6 in, 1 out]
      n283 = call "Draw Overlay Point.vi"("Color"=w577, "Cluster"=w566, "Refnum in"=w586) -> ("Refnum out"=w585:T2)  [unwired: 8 in]
      n284 = call "Draw Overlay Point.vi"("Color"=w577, "Cluster"=w565, "Refnum in"=w585) -> ("Refnum out"=w580:T2)  [unwired: 8 in]
      n285 = Unbundle(w566) -> ("Position.X"=w575:dbl, "Position.Y"=w572:dbl)
      n286 = Unbundle(w565) -> ("P2.X"=w573:dbl, "P2.Y"=w574:dbl)
      n287 = Add(x=w575, y=w573) -> (x+y=w571:dbl)
      n288 = Add(x=w572, y=w574) -> (x+y=w570:dbl)
      n289 = call "IMAQ Overlay Line"("Color"=w577, "End Point"=w565, "Start Point"=w566, "Image"=w580) -> ("Image Out"=w579:T2)  [unwired: 6 in, 1 out]
      n290 = Divide(x=w571, y=w569) -> (x/y=w568:dbl)
      n291 = Divide(x=w570, y=w569) -> (x/y=w567:dbl)
      n292 = Bundle(w568, w567) -> (w564:cluster{dbl, dbl})  [unwired: 1 in]
      n293 = call "IMAQ Overlay Text"("Text Color (black)"=w577, "String"="Caliper", "Origin"=w564, "Image"=w579) -> ("Image Out"=w578:T2)  [unwired: 6 in, 1 out]
    }
    frame 9 {
      w626 = 2.0 ("y")
      # "輸出中線"
      # "Mid Line尋找點與線中間的中線"
      n294 = Unbundle By Name(w646) -> ("Result.Position.X"=w641:dbl, "Result.Position.Y"=w640:dbl, "Result.P2.X"=w639:dbl, "Result.P2.Y"=w638:dbl)
      n295 = Array Subset(array=w648, length=4) -> (w649:T5[])  [unwired: 1 in]
      n296 = for {
        tunnel: w649 -> [w663] mode=indexing
        tunnel: w647 -> [w661]
        shift-right: [w656] -> w643
        shift-left: w645 -> [w659]
        tunnel: [w652] -> w634
        tunnel: [w651] -> w644 mode=indexing
        i -> [w655]
        w652 = u32 16711680 ("Text Color (black)")
        # "輸入第一點與第二點為直線第三點為中點"
        n297 = Unbundle By Name(w663) -> ("Type"=w662:T6, "Index"=w660:i32)
        n298 = Increment(x=w655) -> (x+1=w653:i32)
        n299 = case shown="\"CaliperResult\"" w662 {
          tunnel: w661 -> [w671 _]
          tunnel: w660 -> [w670 _]
          tunnel: [w666 _] -> w651
          tunnel: [FALSE ("StepError?") _] -> _
          tunnel: w659 -> [w664 w672]
          tunnel: [w664 w672] -> w658
          frame "AnalysisResult", Default {
            n300 = Index Array(array=w671, index=w670) -> (element=w669:T1)
            n301 = Unbundle By Name(w669) -> ("Position_X"=w668:dbl, "Position_Y"=w667:dbl)
            n302 = Bundle("Position_X"=w668, "Position_Y"=w667) -> (w666:cluster{"Position_X":dbl, "Position_Y":dbl})  [unwired: 1 in]
          }
          frame "CaliperResult" {
          }
        }
        n303 = Number To Decimal String(number=w653) -> (decimal integer string=w654:string)  [unwired: 1 in]
        n304 = call "Draw Overlay Point.vi"("Color"=w652, "Cluster"=w651, "Refnum in"=w658) -> ("Refnum out"=w657:T2)  [unwired: 8 in]
        n305 = call "IMAQ Overlay Text"("Text Color (black)"=w652, "String"=w654, "Origin"=w651, "Image"=w657) -> ("Image Out"=w656:T2)  [unwired: 6 in, 1 out]
      }
      n306 = Bundle("P2.X"=w639, "P2.Y"=w638) -> (w622:cluster{"P2.X":dbl, "P2.Y":dbl})  [unwired: 1 in]
      n307 = Bundle("Position.X"=w641, "Position.Y"=w640) -> (w623:cluster{"Position.X":dbl, "Position.Y":dbl})  [unwired: 1 in]
      n308 = Index Array(array=w644) -> (element #1=w620:cluster{"Position_X":dbl, "Position_Y":dbl}, element #2=w619:cluster{"Position_X":dbl, "Position_Y":dbl})  [unwired: 2 in]
      n309 = call "IMAQ Overlay Line"("Color"=w634, "End Point"=w619, "Start Point"=w620, "Image"=w643) -> ("Image Out"=w618:T2)  [unwired: 6 in, 1 out]
      n310 = call "Draw Overlay Point.vi"("Color"=w634, "Cluster"=w623, "Refnum in"=w618) -> ("Refnum out"=w642:T2)  [unwired: 8 in]
      n311 = call "Draw Overlay Point.vi"("Color"=w634, "Cluster"=w622, "Refnum in"=w642) -> ("Refnum out"=w637:T2)  [unwired: 8 in]
      n312 = Unbundle(w623) -> ("Position.X"=w632:dbl, "Position.Y"=w629:dbl)
      n313 = Unbundle(w622) -> ("P2.X"=w630:dbl, "P2.Y"=w631:dbl)
      n314 = Add(x=w632, y=w630) -> (x+y=w628:dbl)
      n315 = Add(x=w629, y=w631) -> (x+y=w627:dbl)
      n316 = call "IMAQ Overlay Line"("Color"=w634, "End Point"=w622, "Start Point"=w623, "Image"=w637) -> ("Image Out"=w636:T2)  [unwired: 6 in, 1 out]
      n317 = Divide(x=w628, y=w626) -> (x/y=w625:dbl)
      n318 = Divide(x=w627, y=w626) -> (x/y=w624:dbl)
      n319 = Bundle(w625, w624) -> (w621:cluster{dbl, dbl})  [unwired: 1 in]
      n320 = call "IMAQ Overlay Text"("Text Color (black)"=w634, "String"="Caliper", "Origin"=w621, "Image"=w636) -> ("Image Out"=w635:T2)  [unwired: 6 in, 1 out]
    }
  }
  n321 = property class="ImageControl"(reference=w7, "Value"=w6) -> ()  [unwired: 1 in, 2 out]
